vi "Controller Load Configuration From Parameters.vi"(8 "error in (no error)":errorcluster, 11 "FOFB Parameters":T1) -> (0 "error out":errorcluster, 3 "FOFB Configuration":T8)   [LabVIEW 2011, in "Controller VIs.lvlib"]
uses:
  Controller VIs.lvlib
  Types Definitions/Type FOFB Configuration.ctl
  Types Definitions/Type FOFB Parameters.ctl
  Types Definitions/Type Network Configuration.ctl
  Types Definitions/Type FA Configuration.ctl
  Types Definitions/Type Response Matrix Measurement Configuration.ctl
  Types Definitions/Type Correction Algorithm Configuration.ctl
  Types Definitions/Type Acquisition Network Configuration.ctl
  Types Definitions/Type Actuation Network Configuration.ctl
  Types Definitions/Type PID Parameters.ctl
  XML VIs.lvlib
  Type Definitions.lvlib
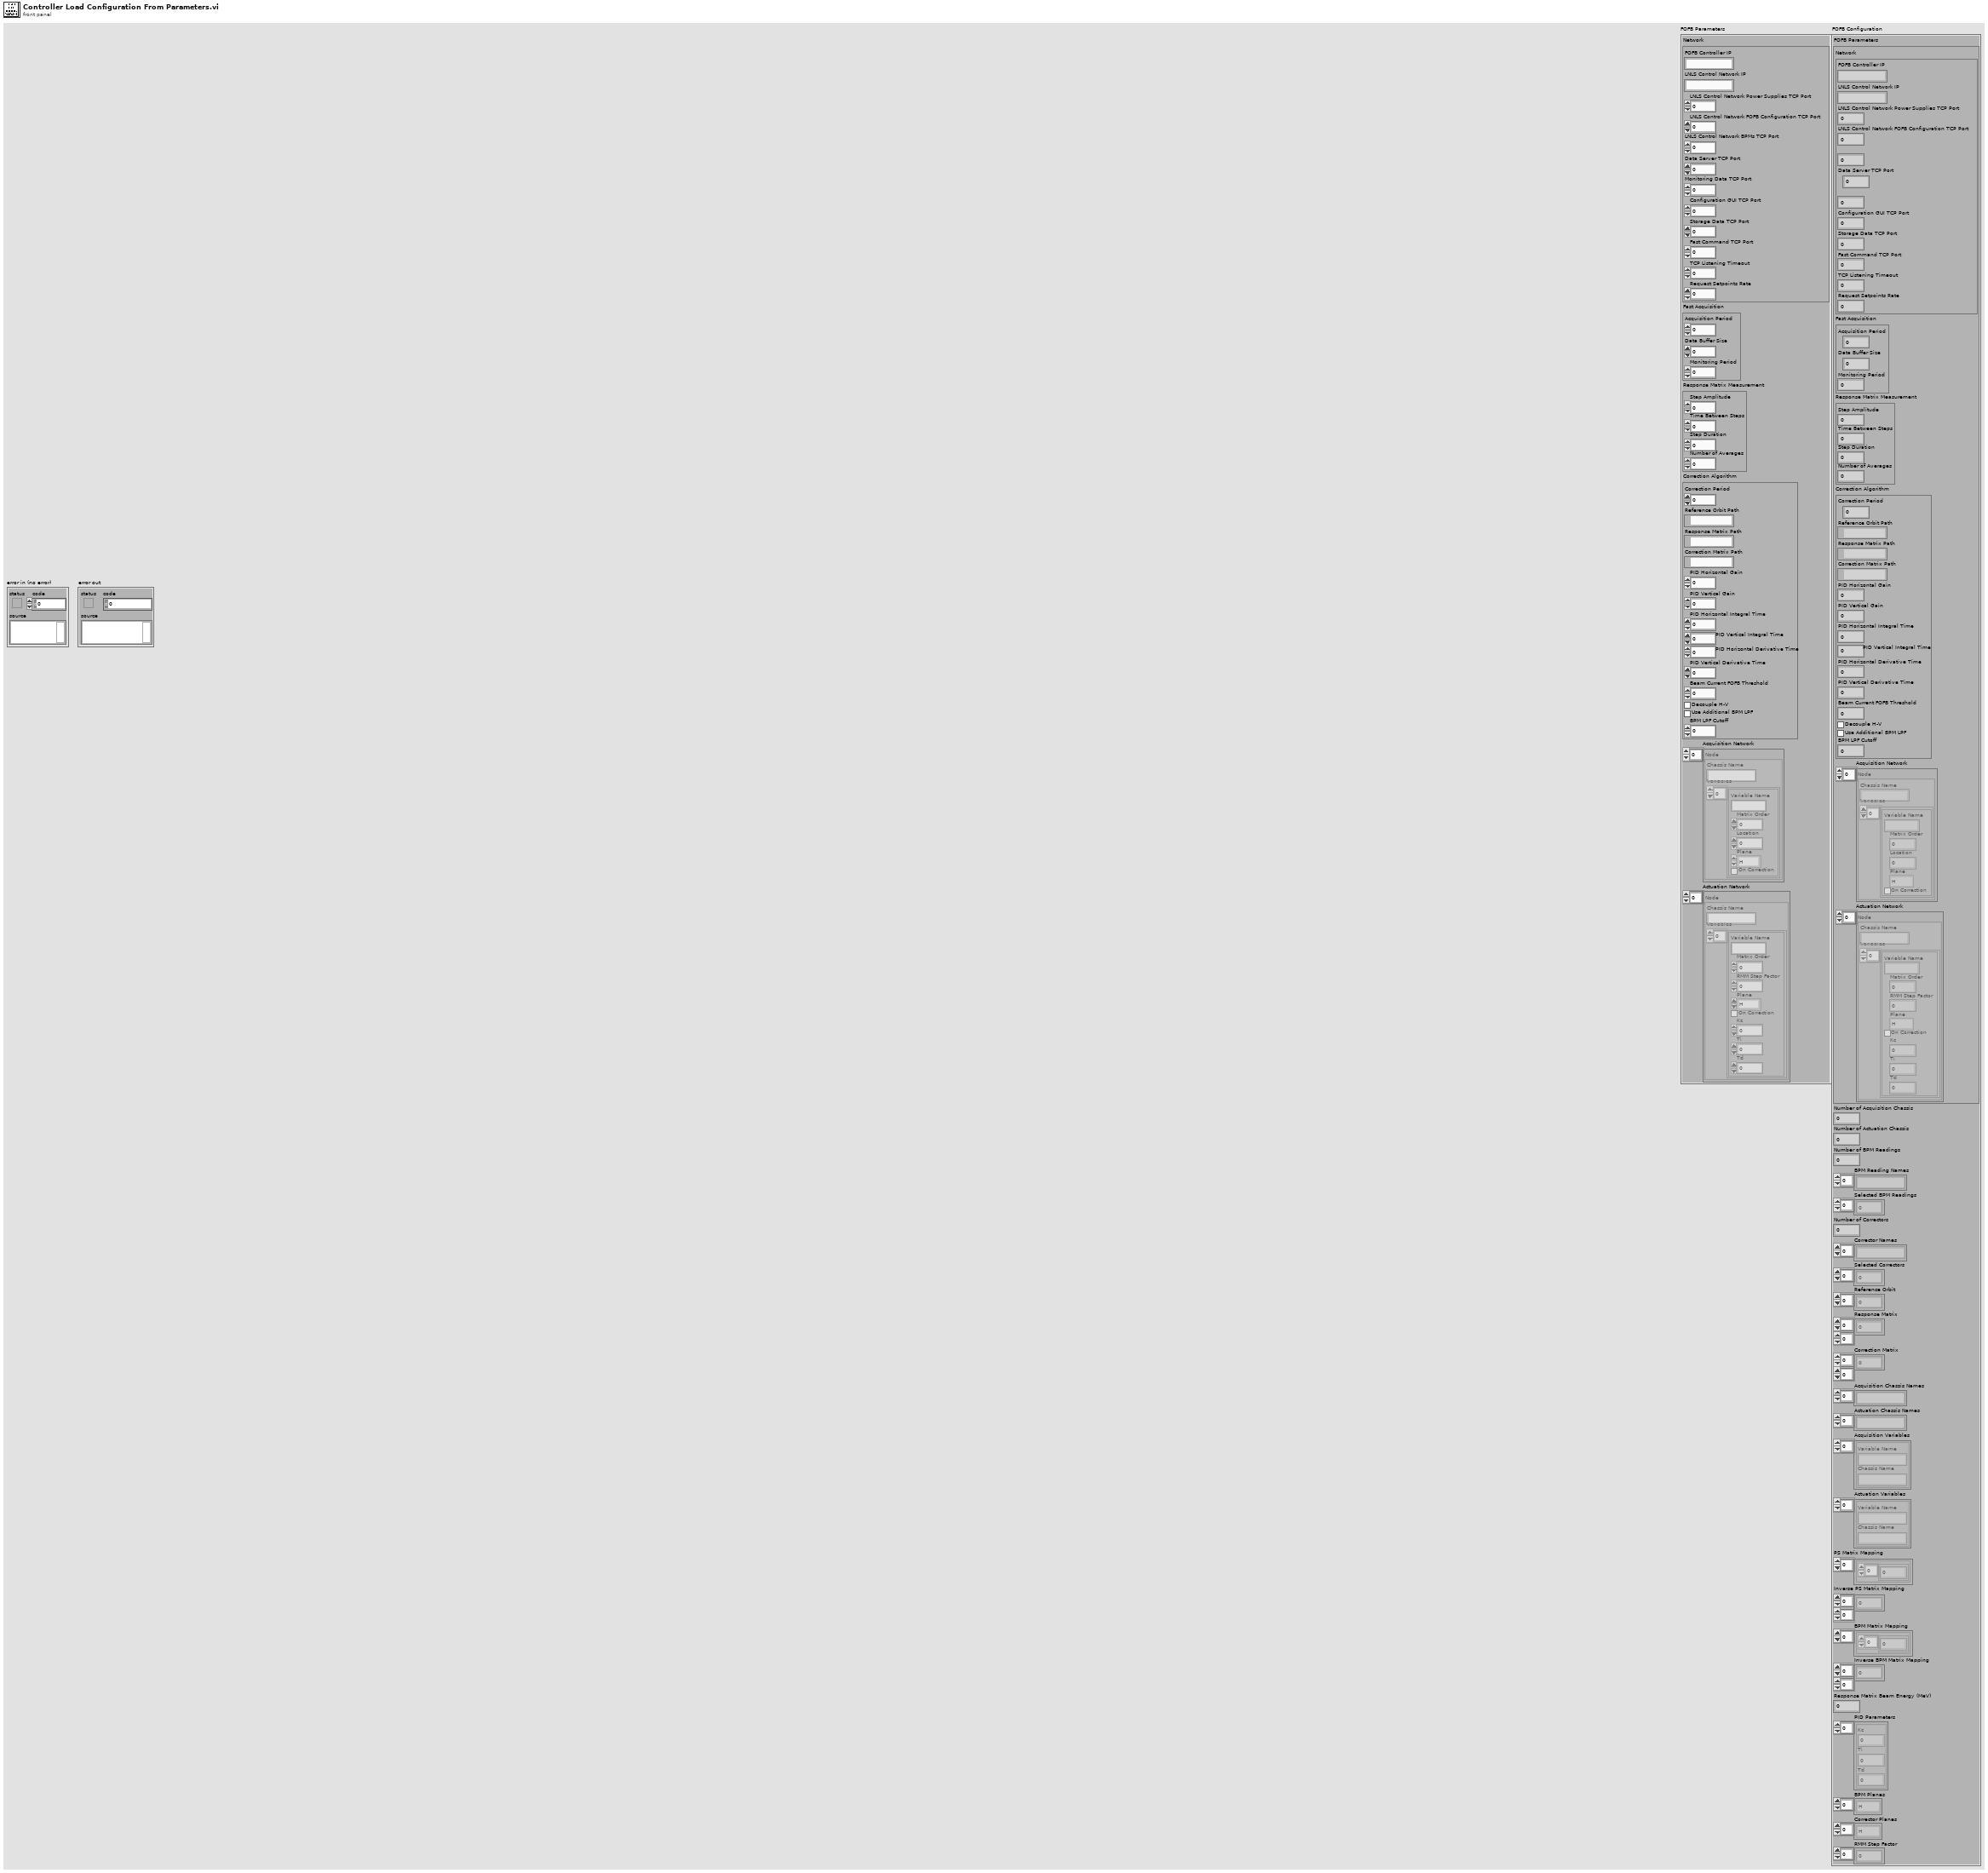
[diagram p1: front panel]
types:
  T1 = typedef "Type Definitions.lvlib/Type FOFB Parameters.ctl" = cluster{"Network":T2, "Fast Acquisition":T3, "Response Matrix Measurement":T4, "Correction Algorithm":T5, "Acquisition Network":T6, "Actuation Network":T7}
  T2 = typedef "Type Definitions.lvlib/Type Network Configuration.ctl" = cluster{"FOFB Controller IP":string, "LNLS Control Network IP":string, "LNLS Control Network Power Supplies TCP Port":u16, "LNLS Control Network FOFB Configuration TCP Port":u16, "LNLS Control Network BPMs TCP Port":u16, "Data Server TCP Port":u16, "Monitoring Data TCP Port":u16, "Configuration GUI TCP Port":u16, "Storage Data TCP Port":u16, "Fast Command TCP Port":u16, "TCP Listening Timeout":i32, "Request Setpoints Rate":u16}
  T3 = typedef "Type Definitions.lvlib/Type FA Configuration.ctl" = cluster{"Acquisition Period":u32, "Data Buffer Size":u32, "Monitoring Period":u32}
  T4 = typedef "Type Definitions.lvlib/Type Response Matrix Measurement Configuration.ctl" = cluster{"Step Amplitude":dbl, "Time Between Steps":u32, "Step Duration":u32, "Number of Averages":u32}
  T5 = typedef "Type Definitions.lvlib/Type Correction Algorithm Configuration.ctl" = cluster{"Correction Period":u32, "Reference Orbit Path":path, "Response Matrix Path":path, "Correction Matrix Path":path, "PID Horizontal Gain":dbl, "PID Vertical Gain":dbl, "PID Horizontal Integral Time":dbl, "PID Vertical Integral Time":dbl, "PID Horizontal Derivative Time":dbl, "PID Vertical Derivative Time":dbl, "Beam Current FOFB Threshold":dbl, "Decouple H-V":bool, "Use Additional BPM LPF":bool, "BPM LPF Cutoff":dbl}
  T6 = typedef "Type Definitions.lvlib/Type Acquisition Network Configuration.ctl" = cluster{"Chassis Name":string, "Variables":cluster{"Variable Name":string, "Matrix Order":u32, "Location":dbl, "Plane":enum8{"H", "V"}, "On Correction":bool}[]}[]
  T7 = typedef "Type Definitions.lvlib/Type Actuation Network Configuration.ctl" = cluster{"Chassis Name":string, "Variables":cluster{"Variable Name":string, "Matrix Order":u32, "RMM Step Factor":dbl, "Plane":enum8{"H", "V"}, "On Correction":bool, "Kc":dbl, "Ti":dbl, "Td":dbl}[]}[]
  T8 = typedef "Type Definitions.lvlib/Type FOFB Configuration.ctl" = cluster{"FOFB Parameters":T1, "Number of Acquisition Chassis":i32, "Number of Actuation Chassis":i32, "Number of BPM Readings":i32, "BPM Reading Names":string[], "Selected BPM Readings":u32[], "Number of Correctors":i32, "Corrector Names":string[], "Selected Correctors":u32[], "Reference Orbit":dbl[], "Response Matrix":dbl[][], "Correction Matrix":dbl[][], "Acquisition Chassis Names":string[], "Actuation Chassis Names":string[], "Acquisition Variables":cluster{"Variable Name":string, "Chassis Name":string}[], "Actuation Variables":cluster{"Variable Name":string, "Chassis Name":string}[], "PS Matrix Mapping":cluster{u32[]}[], "Inverse PS Matrix Mapping":u32[][], "BPM Matrix Mapping":cluster{u32[]}[], "Inverse BPM Matrix Mapping":u32[][], "Response Matrix Beam Energy (MeV)":dbl, "PID Parameters":T9[], "BPM Planes":enum8{"H", "V"}[], "Corrector Planes":enum8{"H", "V"}[], "RMM Step Factor":dbl[]}
  T9 = typedef "Type Definitions.lvlib/Type PID Parameters.ctl" = cluster{"Kc":fxp<+/-,16,8>, "Ti":fxp<+/-,16,8>, "Td":fxp<+/-,16,8>}
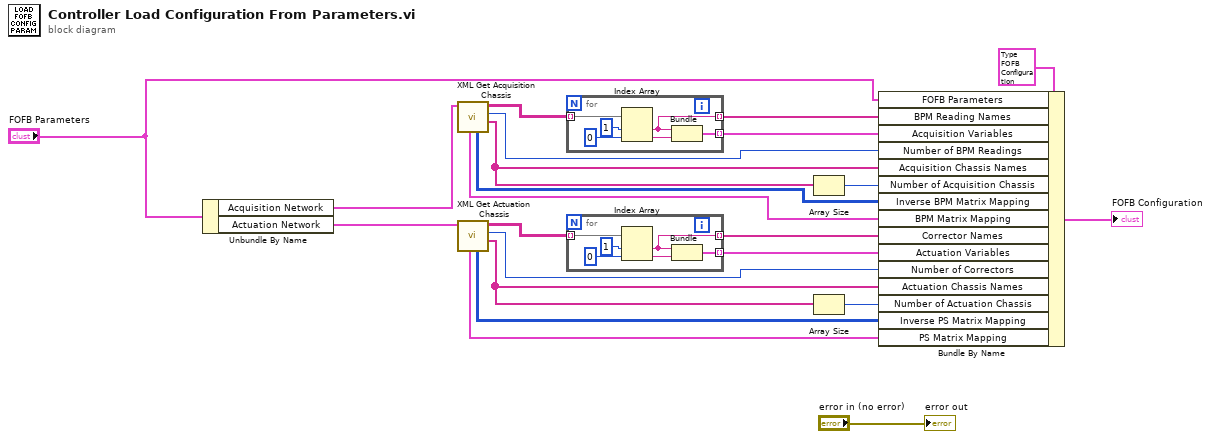
[diagram p0: block diagram]
diagram:
  n1 = Unbundle By Name("FOFB Parameters") -> ("Acquisition Network"=w2:T6, "Actuation Network"=w1:T7)
  n2 = call "XML Get Acquisition Chassis.vi"("Acquisition Network"=w2) -> ("Acquisition Chassis Names"=w11:string[], "Number of BPM Readings"=w17:i32, "Acquisition Variable Names"=w12:string[][], "Inverse BPM Matrix Mapping"=w20:u32[][], "BPM Matrix Mapping"=w21:cluster{u32[]}[])  [unwired: 4 in, 2 out]
  n3 = call "XML Get Actuation Chassis.vi"("Actuation Network"=w1) -> ("Actuation Chassis Names"=w7:string[], "Number of Correctors"=w15:i32, "Actuation Variable Names"=w5:string[][], "Inverse PS Matrix Mapping"=w8:u32[][], "PS Matrix Mapping"=w19:cluster{u32[]}[])  [unwired: 3 in, 3 out]
  n4 = for {
    tunnel: w12 -> [w27] mode=indexing
    tunnel: [w26] -> w14 mode=indexing
    tunnel: [w23] -> w13 mode=indexing
    n5 = Index Array(array=w27, index #1=1 ("index"), index #2=0 ("index")) -> (element #1=w23:string, element #2=w25:string)
    n6 = Bundle(w23, w25) -> (w26:cluster{string, string})  [unwired: 1 in]
  }
  n7 = for {
    tunnel: w5 -> [w33] mode=indexing
    tunnel: [w32] -> w6 mode=indexing
    tunnel: [w29] -> w10 mode=indexing
    n8 = Index Array(array=w33, index #1=1 ("index"), index #2=0 ("index")) -> (element #1=w29:string, element #2=w31:string)
    n9 = Bundle(w29, w31) -> (w32:cluster{string, string})  [unwired: 1 in]
  }
  n10 = Array Size(array=w11) -> (size(s)=w4:i32)
  n11 = Array Size(array=w7) -> (size(s)=w18:i32)
  n12 = Bundle By Name(cluster=T8 {"FOFB Parameters"={"Network"={"FOFB Controller IP"="", "LNLS Control Network IP"="", "LNLS Control Network Power Supplies TCP Port"=0, "LNLS Control Network FOFB Configuration TCP Port"=0, "LNLS Control Network BPMs TCP Port"=0, "Data Server TCP Port"=0, "Monitoring Data TCP Port"=0, "Configuration GUI TCP Port"=0, "Storage Data TCP Port"=0, "Fast Command TCP Port"=0, "TCP Listening Timeout"=0, "Request Setpoints Rate"=0}, "Fast Acquisition"={"Acquisition Period"=0, "Data Buffer Size"=0, "Monitoring Period"=0}, "Response Matrix Measurement"={"Step Amplitude"=0.0, "Time Between Steps"=0, "Step Duration"=0, "Number of Averages"=0}, "Correction Algorithm"={"Correction Period"=0, "Reference Orbit Path"=path "", "Response Matrix Path"=path "", "Correction Matrix Path"=path "", "PID Horizontal Gain"=0.0, "PID Vertical Gain"=0.0, "PID Horizontal Integral Time"=0.0, "PID Vertical Integral Time"=0.0, "PID Horizontal Derivative Time"=0.0, "PID Vertical Derivative Time"=0.0, "Beam Current FOFB Threshold"=0.0, "Decouple H-V"=FALSE, "Use Additional BPM LPF"=FALSE, "BPM LPF Cutoff"=0.0}, "Acquisition Network"=[], "Actuation Network"=[]}, "Number of Acquisition Chassis"=0, "Number of Actuation Chassis"=0, "Number of BPM Readings"=0, "BPM Reading Names"=[], "Selected BPM Readings"=[], "Number of Correctors"=0, "Corrector Names"=[], "Selected Correctors"=[], "Reference Orbit"=[], "Response Matrix"=[], "Correction Matrix"=[], "Acquisition Chassis Names"=[], "Actuation Chassis Names"=[], "Acquisition Variables"=[], "Actuation Variables"=[], "PS Matrix Mapping"=[], "Inverse PS Matrix Mapping"=[], "BPM Matrix Mapping"=[], "Inverse BPM Matrix Mapping"=[], "Response Matrix Beam Energy (MeV)"=0.0, "PID Parameters"=[], "BPM Planes"=[], "Corrector Planes"=[], "RMM Step Factor"=[]}, "FOFB Parameters"="FOFB Parameters", "BPM Reading Names"=w13, "Acquisition Variables"=w14, "Number of BPM Readings"=w17, "Acquisition Chassis Names"=w11, "Number of Acquisition Chassis"=w4, "Inverse BPM Matrix Mapping"=w20, "BPM Matrix Mapping"=w21, "Corrector Names"=w10, "Actuation Variables"=w6, "Number of Correctors"=w15, "Actuation Chassis Names"=w7, "Number of Actuation Chassis"=w18, "Inverse PS Matrix Mapping"=w8, "PS Matrix Mapping"=w19) -> (→"FOFB Configuration":T8)
  "error out" <- "error in (no error)"
